vi "CONTINEOUS READ CAN.vi"(0 "interface":string(combo)="CAN0", 2 "Baudrate":u32=500000, 5 "WRITE CMD":u8[](array[numeric]) format="%.0x", 6 "Error in 2":errorcluster {"code" format="%.0x"}, 8 "Default 3":string, 9 "Default ID 1":string="20000687", 10 "CAN OPERATION":T2, 11 "WRITE AR ID":u32 format="%.0x", 13 "DataLength":u32=8, 15 "Default ID 2":string="20000688") -> (3 "ArbitrationId 2":u32 format="%.0x", 12 "Data":u8[](array[numeric]), 16 "ActualDataSize (Frames)":u32, 17 "Actual CAN Array":string[][](array[string]), 22 "CAN DATA":T1[](array[typedef]) {"Data" format="%.0x"; "ArbitrationId" format="%.0x"; "Timestamp" format="%<%I:%M:%S%3u %p\n%m/%d/%Y>T"}, 25 "can read array":u32[][](array[numeric]), 26 "Error out 2":errorcluster {"code" format="%.0x"})   [LabVIEW 2017]
uses:
  CAN_OPERATION _TYPEDEF.ctl
  <vilib>/nican/nican.llb/CanFrameTimed.ctl
  <vilib>/nican/nican.llb/xobjhandle.ctl
  <vilib>/nican/nican.llb/ncNetAttr.ctl
  d29f5f51-2dbb-4be0-bfac-dc6a67a75a0a.vi
  ef5e345f-b127-46e6-b386-8f45186839bc.vi
  bcc05463-866b-46b8-b575-a31bcf1911b9.vi
  6277f388-f3ac-4f71-9de4-5b592c734c63.vi
panel:
  out "Output Array":string[][](array[string])
  out "ActualDataSize (Frames) 2":u32
  out "ArbitrationId 3":u32 format="%.0x"
  out "initialized array":string[][](array[string])
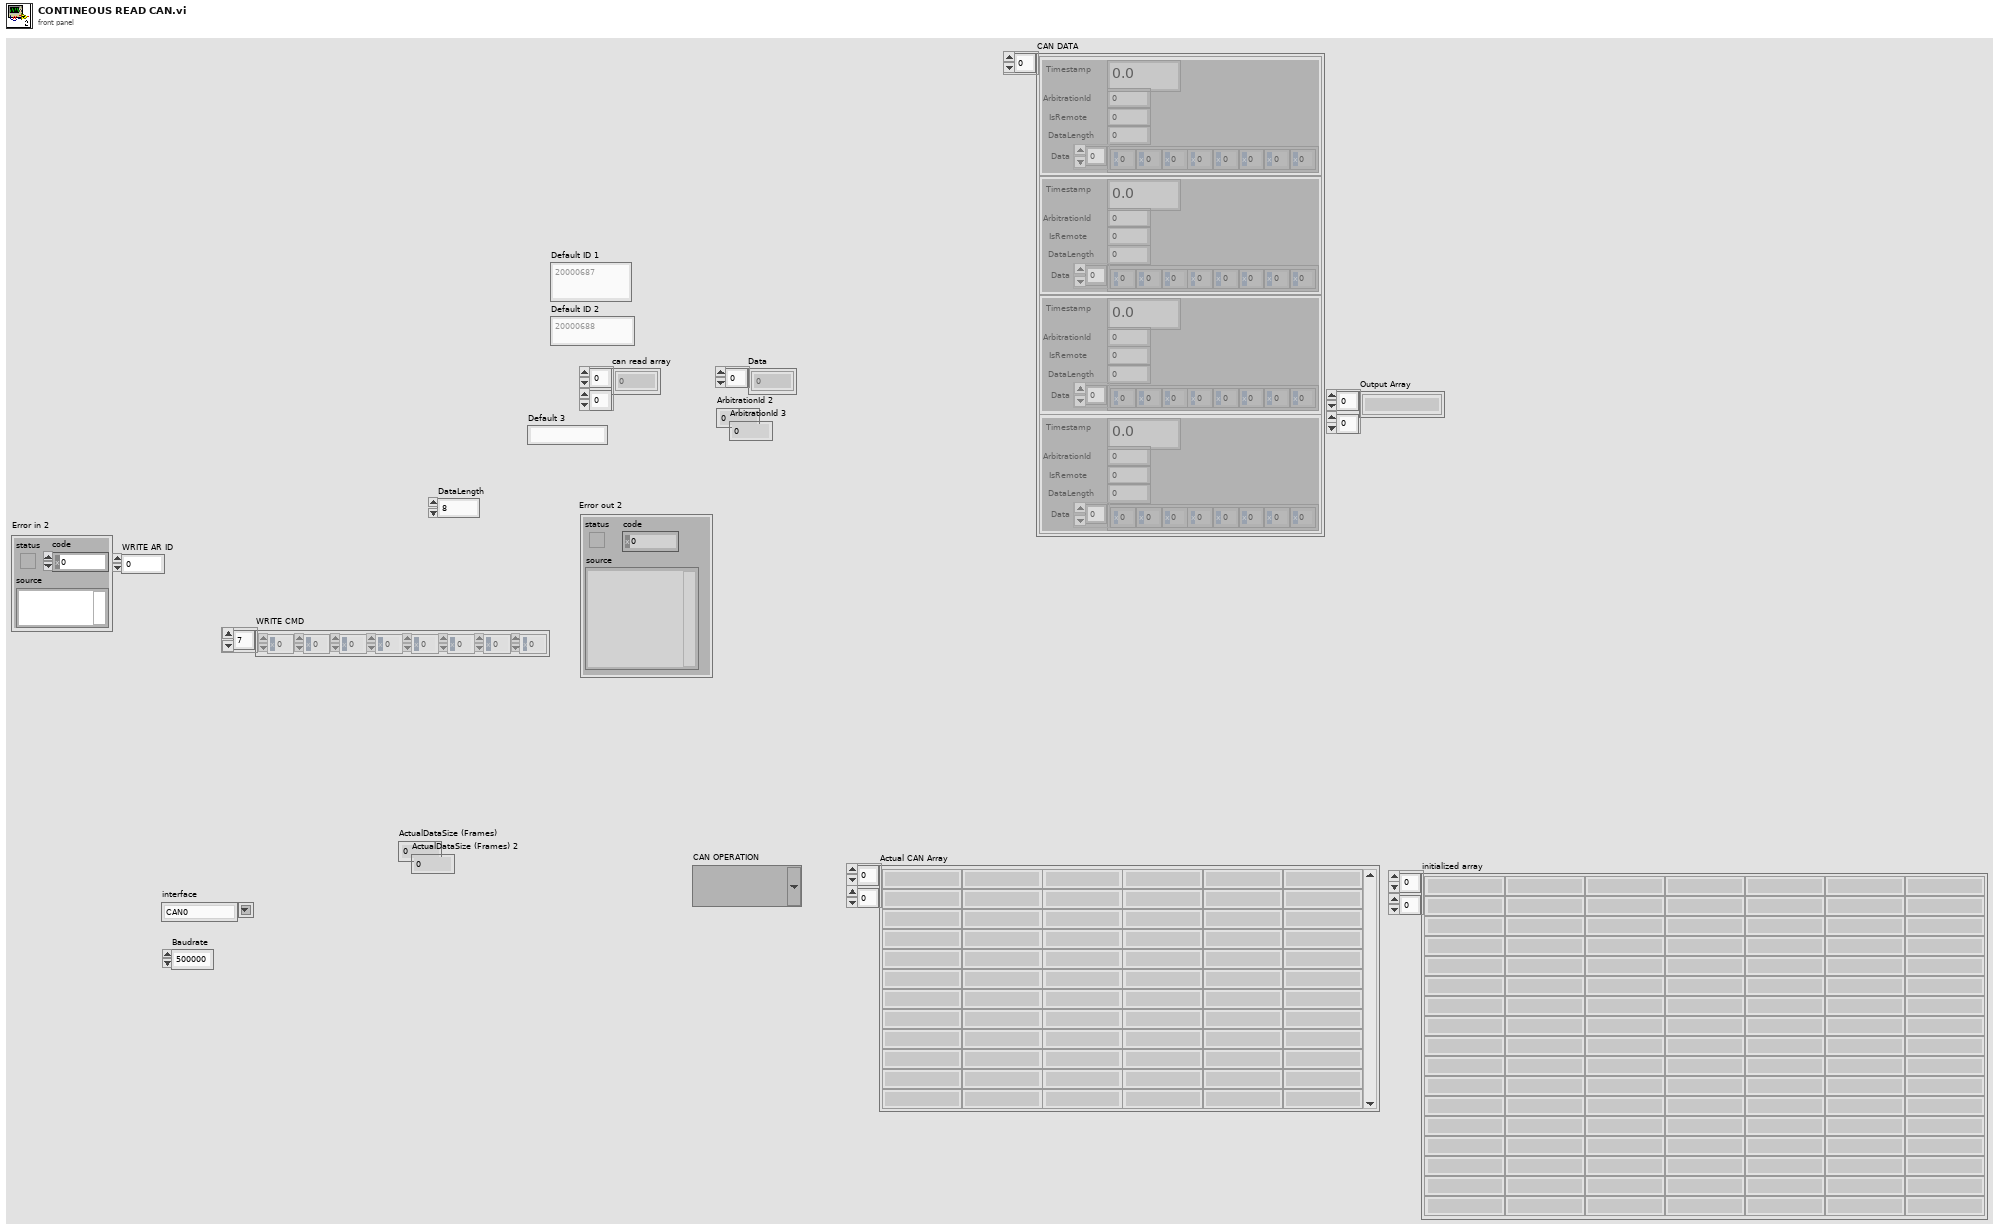
[diagram p1: front panel]
types:
  T1 = typedef "CanFrameTimed.ctl" = cluster{"Timestamp":dbl, "ArbitrationId":u32, "IsRemote":u8, "DataLength":u8, "Data":u8[]}
  T2 = typedef "CAN_OPERATION _TYPEDEF.ctl" = string
  T3 = typedef "xobjhandle.ctl" = u32
  T4 = cluster{"Baudrate":u32, "interface":string, "ObjHandle out":T3, "CAN DATA":T1[], "Data":u32[], "can read array":u32[][], "Actual CAN Array":string[][], "Default ID 1":string, "Default ID 2":string}
  T5 = typedef "ncNetAttr.ctl" = cluster{"Start On Open":enum32{"FALSE", "TRUE"}, "Baud Rate":u32, "Read Queue Length":u32, "Write Queue Length":u32, "Standard Comparator":u32, "Standard Mask":u32, "Extended Comparator":u32, "Extended Mask":u32}
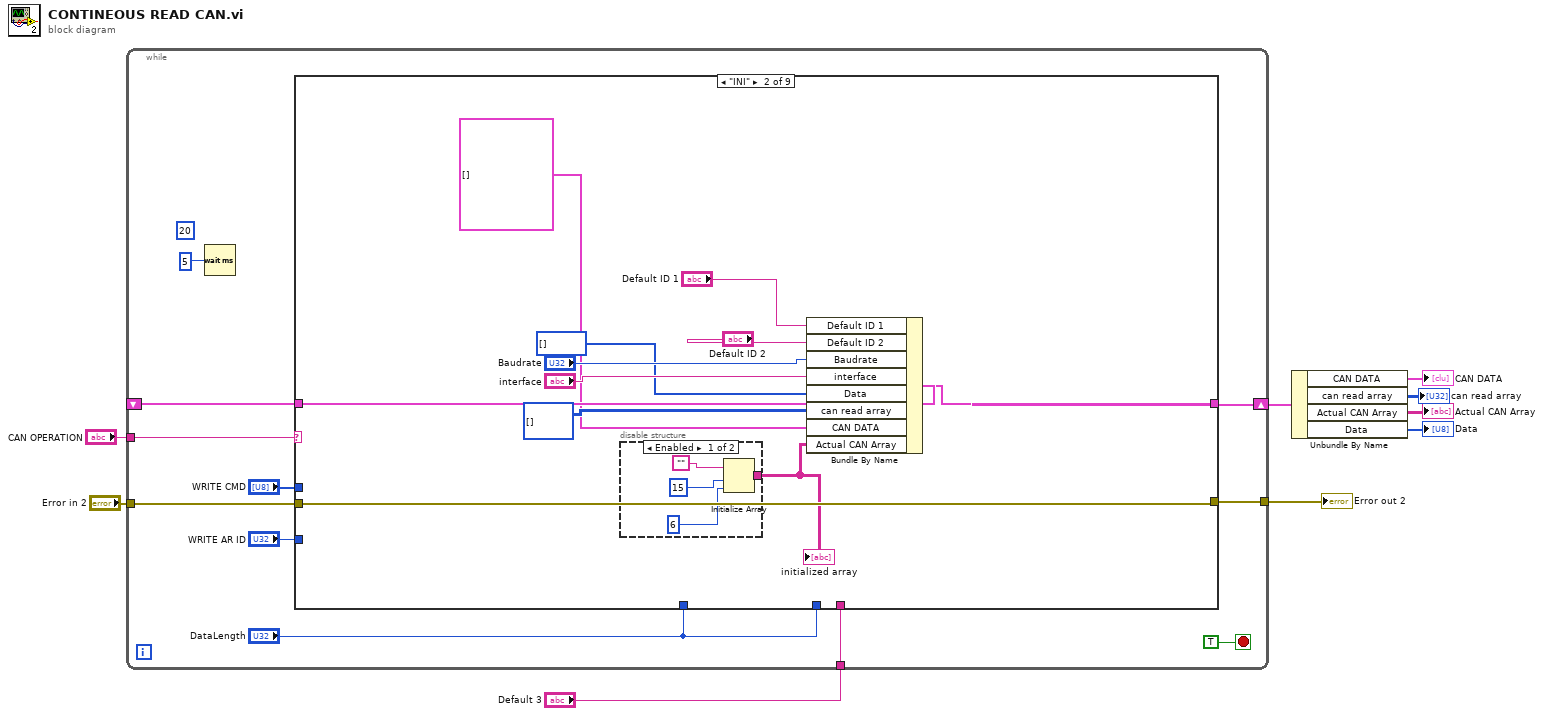
[diagram p0: block diagram]
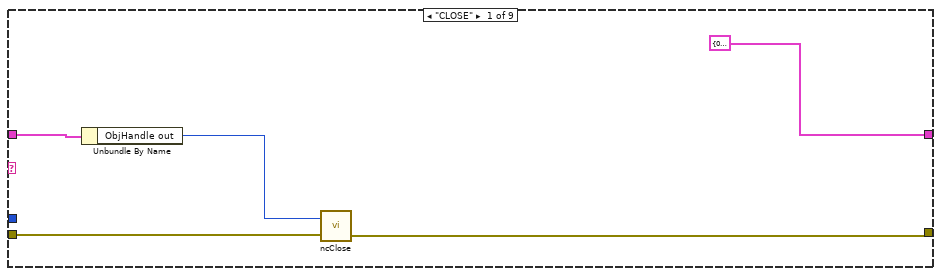
[diagram p2: hidden frame]
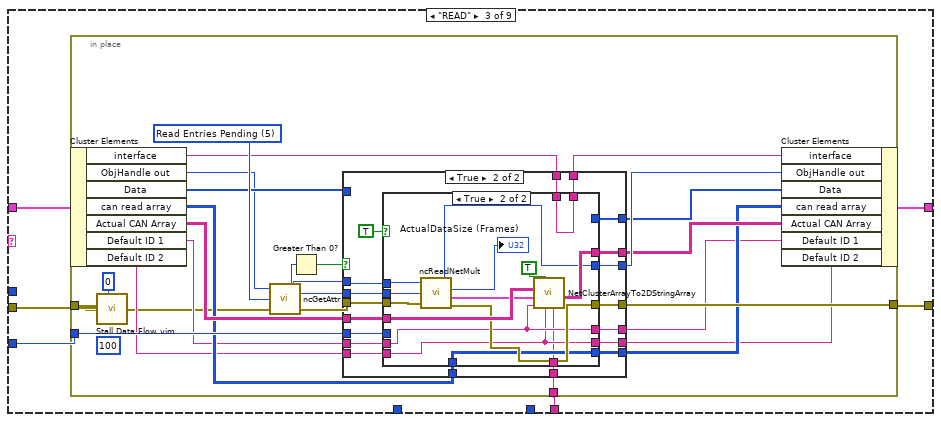
[diagram p4: hidden frame]
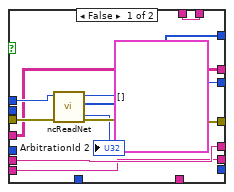
[diagram p6: hidden frame]
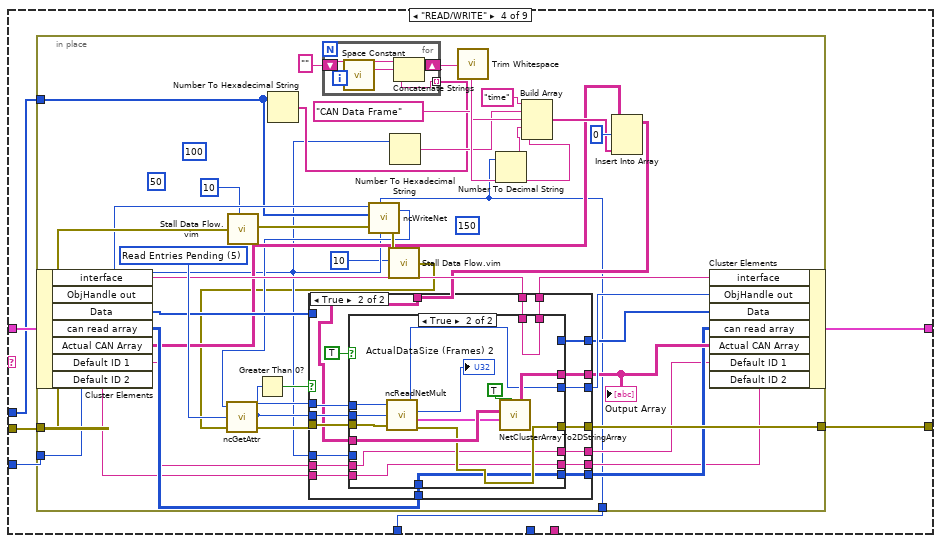
[diagram p7: hidden frame]
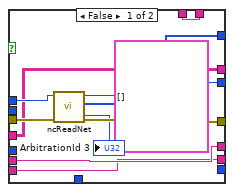
[diagram p9: hidden frame]
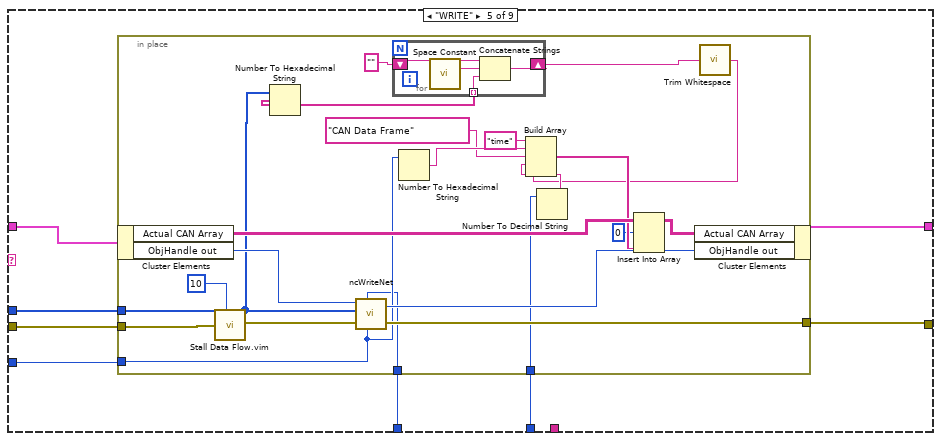
[diagram p10: hidden frame]
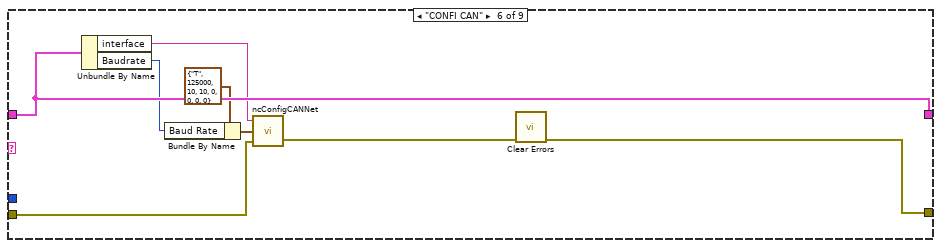
[diagram p11: hidden frame]
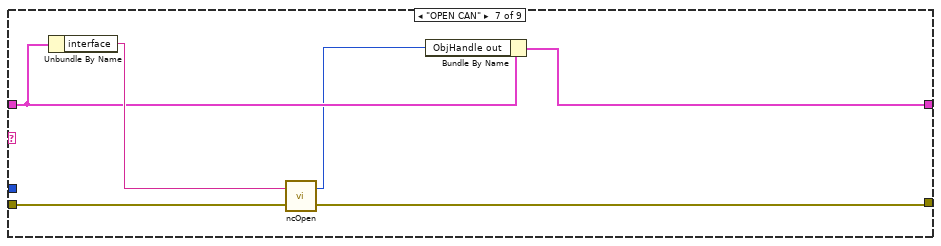
[diagram p12: hidden frame]
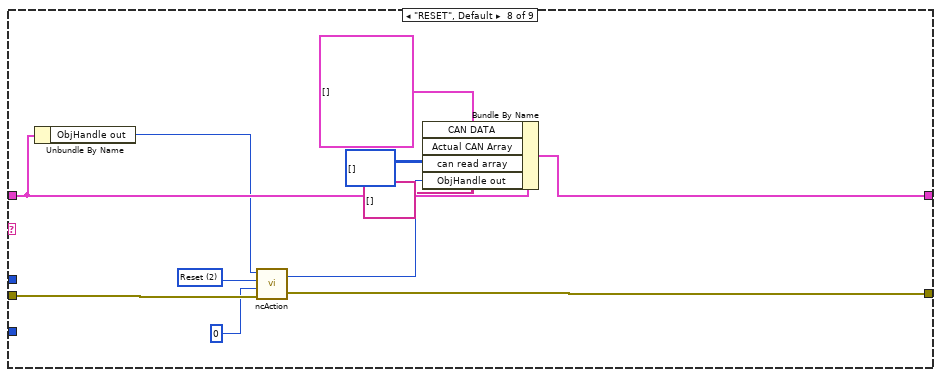
[diagram p13: hidden frame]
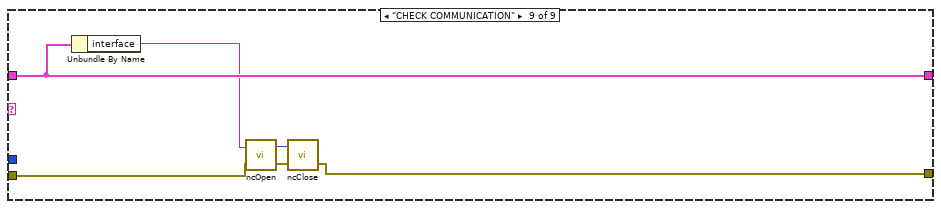
[diagram p14: hidden frame]
diagram:
  n1 = while {
    tunnel: "CAN OPERATION" -> [w20]
    tunnel: [w18] -> w2
    tunnel: "Error in 2" -> [w17]
    shift-right: [w15] -> w7
    shift-left: _ -> [w16]
    tunnel: "Default 3" -> [w10]
    stop <- TRUE stop-if-true
    (unwired) u32 20 ("millisecond multiple")
    n2 = Wait (ms)(milliseconds to wait=u32 5 ("millisecond multiple")) -> ()  [unwired: 1 out]
    n3 = case shown="\"INI\"" w20 {
      tunnel: [w24 w32 w42 w125 w229 w257 w265 w278 w285] -> w18
      tunnel: w17 -> [w25 w32 w46 w129 w230 w262 w269 w277 w282]
      tunnel: w16 -> [w23 w36 w45 w128 w225 w264 w268 w281 w284]
      tunnel: [T4 {"Baudrate"=0, "interface"="", "ObjHandle out"=0, "CAN DATA"=[], "Data"=[], "can read array"=[[710, 1, 0, 0, 0, 0, 0, 0, 0], [711, 255, 255, 255, 255, 0, 0, 0, 0], [712, 0, 0, 0, 0, 0, 0, 0, 0], [712, 0, 0, 0, 0, 0, 0, 0, 0], [720, 136, 2, 27, 96, 16, 0, 0, 0], [722, 24, 0, 0, 123, 100, 131, 12, 107], [723, 0, 0, 187, 131, 74, 4, 0, 0], [723, 0, 0, 187, 131, 74, 4, 0, 0], [725, 255, 255, 159, 111, 255, 255, 0, 0], [725, 255, 255, 159, 111, 255, 255, 0, 0], [727, 255, 255, 255, 255, 255, 29, 0, 0], [946, 144, 0, 0, 192, 192, 15, 0, 51], [1168, 197, 0, 0, 0, 0, 0, 0, 0], [1168, 197, 0, 0, 0, 0, 0, 0, 0], [1169, 0, 0, 0, 0, 0, 0, 0, 0], [1169, 0, 0, 0, 0, 0, 0, 0, 0], [1280, 0, 0, 0, 0, 0, 0, 0, 0]], "Actual CAN Array"=[["05:30:00.000", "         0", "CAN Data Frame\r\n", " 0", "No Data\r\n"], ["05:30:00.000", "         0", "CAN Data Frame\r\n", " 0", "No Data\r\n"]], "Default ID 1"="", "Default ID 2"=""} w33 w44 w127 w228 w264 w266 w280 w284] -> w15
      tunnel: "WRITE CMD" -> [_ _ _ w124 w226 _ _ _ _]
      tunnel: "WRITE AR ID" -> [_ _ w43 w126 w227 _ _ _ _]
      tunnel: "DataLength" -> [_ _ _ _ w224 _ _ _ _]
      tunnel: "DataLength" -> [_ _ _ w123 w223 _ _ _ _]
      tunnel: w10 -> [_ _ w41 _ _ _ _ _ _]
      frame "CLOSE" {
        n4 = Unbundle By Name(w23) -> ("ObjHandle out"=w22:T3)
        n5 = call <vilib>:"ncClose.vi"("Error in"=w25, "ObjHandle in"=w22) -> ("Error out"=w24:errorcluster)  [unwired: 1 in]
      }
      frame "INI" {
        n6 = disable-structure shown="Enabled" {
          disable-tunnel: [w38 _] -> w28
          frame Enabled {
            n7 = Initialize Array("", 15, 6) -> (w38:string[][])
          }
          frame Disabled {
          }
        }
        "initialized array" <- w28
        n8 = Bundle By Name(cluster=w36, "Default ID 1"="Default ID 1", "Default ID 2"="Default ID 2", "Baudrate"="Baudrate", "interface"="interface", "Data"=u8[] [], "can read array"=u32[][] [], "CAN DATA"=T1[] [], "Actual CAN Array"=w28) -> (w33:T4)
      }
      frame "READ" {
        n9 = in-place {
          in-place-border: w46 -> [w58]
          in-place-border: w43 -> [w67]
          in-place-border: [w56] -> w42
          in-place-border: w41 -> [w47]
          (unwired) u32 100 ("millisecond multiple")
          w71 = u32 5 items=["(reserved)", "Protocol Version", "Software Version", "Object State", "(reserved)", "Read Entries Pending", "Write Entries Pending", "ReadMult Size for Notification", "Listen Only?", "Self Reception?", "Transmit Error Counter", "Receive Error Counter", "Single Shot Transmit?", "Series 2 Filter Mode", "Series 2 Mask", "Series 2 Comparator", "Serial Number", "Form Factor", "Series", "Transceiver Type", "Interface Number", "Series 2 Error/Arb Capture", "Transceiver Mode", "Transceiver External Outputs", "Transceiver External Inputs", "Start Trigger Behavior", "Log Comm Warnings", "User RTSI Frame", "Transmit Mode", "Log Start Trigger?", "Timestamp Format", "Master Timebase Rate", "Virtual Bus Timing"] ("AttrId")
          n10 = in-place-cluster #1(w45) -> ("interface"=w65:string, "ObjHandle out"=w57:T3, "Data"=w61:u32[], "can read array"=w55:u32[][], "Actual CAN Array"=w62:string[][], "Default ID 1"=w53:string, "Default ID 2"=w52:string)
          n11 = call "Stall Data Flow.vim"("value in"=w58, "milliseconds to wait"=u32 0 ("millisecond multiple")) -> ("value out"=w49:errorcluster)  [unwired: 1 out]
          n12 = call <vilib>:"ncGetAttr.vi"("Error in"=w49, "AttrId"=w71, "ObjHandle in"=w57) -> ("Error out"=w59:errorcluster, "AttrValue"=w60:u32, "ObjHandle out"=w69:T3)
          n13 = Greater Than 0?(x=w60) -> (x > 0?=w70:bool)
          n14 = case shown="True" w70 {
            tunnel: w59 -> [w77 w97]
            tunnel: [w77 w86] -> w56
            tunnel: w69 -> [w78 w96]
            tunnel: [w78 w95] -> w68
            tunnel: w67 -> [_ w93]
            tunnel: [w74 w92] -> w66
            tunnel: w65 -> [w76 w91]
            tunnel: [w76 w90] -> w64
            tunnel: [w75 w89] -> w63
            tunnel: w62 -> [w75 w88]
            tunnel: w61 -> [w74 _]
            tunnel: w60 -> [_ w87]
            tunnel: w55 -> [_ w85]
            tunnel: [_ w84] -> w54
            tunnel: w53 -> [w73 w83]
            tunnel: w52 -> [w72 w82]
            tunnel: [w73 w81] -> w51
            tunnel: [w72 w80] -> w50
            tunnel: w47 -> [_ w79]
            frame False {
            }
            frame True {
              n15 = case shown="True" TRUE {
                tunnel: w97 -> [w107 w121]
                tunnel: [w106 w113] -> w86
                tunnel: w96 -> [w105 w114]
                tunnel: [w104 w117] -> w95
                tunnel: w93 -> [_ _]
                tunnel: [w102 _] -> w92
                tunnel: w91 -> [w103 w116]
                tunnel: [w103 w116] -> w90
                tunnel: [w100 w120] -> w89
                tunnel: w88 -> [w100 w119]
                tunnel: w87 -> [_ w115]
                tunnel: w85 -> [_ w111]
                tunnel: [_ w111] -> w84
                tunnel: w83 -> [w99 w110]
                tunnel: w82 -> [w98 w109]
                tunnel: [w99 w110] -> w81
                tunnel: [w98 w109] -> w80
                tunnel: w79 -> [_ w108]
                frame False {
                  (unwired) T1[] [] ("101 Array")
                  n16 = call <vilib>:"ncReadNet.vi"("ObjHandle in"=w105, "Error in"=w107) -> ("ArbitrationId"=→"ArbitrationId 2":u32, "ObjHandle out"=w104:T3, "Data"=w102:u8[], "Error out"=w106:errorcluster)  [unwired: 2 in, 3 out]
                }
                frame True {
                  n17 = call <vilib>:"ncReadNetMult.vi"("ObjHandle in"=w114, "Requested Number of Frames"=w115, "Error in"=w121) -> ("ObjHandle out"=w117:T3, "ActualDataSize (Frames)"=→"ActualDataSize (Frames)":u32, "Data"=w112:T1[], "Error out"=w113:errorcluster)
                  n18 = call <vilib>:"NetClusterArrayTo2DStringArray.vi"("Default 2"=w108, "Default 3"=w109, "Hexadecimal?"=TRUE, "Default 1"=w110, "Data from ncReadNetMult"=w112, "Input Array"=w119) -> ("Output Array"=w120:string[][])  [unwired: 5 in]
                }
              }
            }
          }
          n19 = in-place-cluster #1("interface"=w64, "ObjHandle out"=w68, "Data"=w66, "can read array"=w54, "Actual CAN Array"=w63, "Default ID 1"=w51, "Default ID 2"=w50) -> (w44:T4)
        }
      }
      frame "READ/WRITE" {
        n20 = in-place {
          in-place-border: w129 -> [w142]
          in-place-border: w126 -> [w133]
          in-place-border: [w159] -> w125
          in-place-border: w124 -> [w134]
          in-place-border: w123 -> [w132]
          (unwired) u32 150 ("milliseconds to wait")
          (unwired) u32 100 ("milliseconds to wait")
          (unwired) u32 50 ("milliseconds to wait")
          w170 = u32 5 items=["(reserved)", "Protocol Version", "Software Version", "Object State", "(reserved)", "Read Entries Pending", "Write Entries Pending", "ReadMult Size for Notification", "Listen Only?", "Self Reception?", "Transmit Error Counter", "Receive Error Counter", "Single Shot Transmit?", "Series 2 Filter Mode", "Series 2 Mask", "Series 2 Comparator", "Serial Number", "Form Factor", "Series", "Transceiver Type", "Interface Number", "Series 2 Error/Arb Capture", "Transceiver Mode", "Transceiver External Outputs", "Transceiver External Inputs", "Start Trigger Behavior", "Log Comm Warnings", "User RTSI Frame", "Transmit Mode", "Log Start Trigger?", "Timestamp Format", "Master Timebase Rate", "Virtual Bus Timing"] ("AttrId")
          n21 = in-place-cluster #2(w128) -> ("interface"=w165:string, "ObjHandle out"=w138:T3, "Data"=w162:u32[], "can read array"=w158:u32[][], "Actual CAN Array"=w139:string[][], "Default ID 1"=w156:string, "Default ID 2"=w155:string)
          n22 = call "Stall Data Flow.vim"("value in"=w142, "milliseconds to wait"=u32 10) -> ("value out"=w143:errorcluster)  [unwired: 1 out]
          n23 = Number To Hexadecimal String(2:w134) -> (0:w135:string[])  [unwired: 1 in]
          n24 = for {
            shift-right: [w173] -> w151
            shift-left: "" -> [w172]
            tunnel: w135 -> [w171] mode=indexing
            n25 = call <vilib>:"Space Constant.vi"() -> ("String"=w174:string)
            n26 = Concatenate Strings(w172, w174, w171) -> (w173:string)
          }
          n27 = call <vilib>:"ncWriteNet.vi"("ArbitrationId"=w133, "DataLength"=w132, "Error in"=w143, "Data"=w134, "ObjHandle in"=w138) -> ("Error out"=w141:errorcluster, "ObjHandle out"=w137:T3)  [unwired: 1 in]
          n28 = call "Stall Data Flow.vim"("value in"=w141, "milliseconds to wait"=u32 10) -> ("value out"=w130:errorcluster)  [unwired: 1 out]
          n29 = call <vilib>:"ncGetAttr.vi"("Error in"=w130, "AttrId"=w170, "ObjHandle in"=w137) -> ("Error out"=w160:errorcluster, "AttrValue"=w161:u32, "ObjHandle out"=w168:T3)
          n30 = Greater Than 0?(x=w161) -> (x > 0?=w169:bool)
          n31 = Number To Hexadecimal String(2:w133) -> (0:w144:string)  [unwired: 1 in]
          n32 = call <vilib>:"Trim Whitespace.vi"("string"=w151) -> ("trimmed string"=w152:string)  [unwired: 1 in]
          n33 = Number To Decimal String(number=w132) -> (decimal integer string=w145:string)  [unwired: 1 in]
          n34 = Build Array("time" ("element"), w144, "CAN Data Frame", w145, w152) -> (w148:string[])
          n35 = Insert Into Array(array=w139, index (row)=0, new element=w148) -> (w140:string[][])  [unwired: 1 in]
          n36 = case shown="True" w169 {
            tunnel: w160 -> [w179 w198]
            tunnel: [w179 w188] -> w159
            tunnel: w168 -> [w180 w197]
            tunnel: [w180 w196] -> w167
            tunnel: w133 -> [_ w194]
            tunnel: [w177 w193] -> w166
            tunnel: w165 -> [w178 w192]
            tunnel: [w178 w191] -> w164
            tunnel: [_ w190] -> w163
            tunnel: w162 -> [w177 _]
            tunnel: w161 -> [_ w189]
            tunnel: w158 -> [_ w187]
            tunnel: [_ w186] -> w157
            tunnel: w156 -> [w176 w185]
            tunnel: w155 -> [w175 w184]
            tunnel: [w176 w183] -> w154
            tunnel: [w175 w182] -> w153
            tunnel: w140 -> [_ w181]
            frame False {
            }
            frame True {
              n37 = case shown="True" TRUE {
                tunnel: w198 -> [w208 w221]
                tunnel: [w207 w213] -> w188
                tunnel: w197 -> [w206 w214]
                tunnel: [w205 w217] -> w196
                tunnel: w194 -> [_ _]
                tunnel: [w203 _] -> w193
                tunnel: w192 -> [w204 w216]
                tunnel: [w204 w216] -> w191
                tunnel: [w201 w220] -> w190
                tunnel: w181 -> [w201 w219]
                tunnel: w189 -> [_ w215]
                tunnel: w187 -> [_ w211]
                tunnel: [_ w211] -> w186
                tunnel: w185 -> [w200 w210]
                tunnel: w184 -> [w199 w209]
                tunnel: [w200 w210] -> w183
                tunnel: [w199 w209] -> w182
                frame False {
                  (unwired) T1[] [] ("101 Array")
                  n38 = call <vilib>:"ncReadNet.vi"("ObjHandle in"=w206, "Error in"=w208) -> ("ArbitrationId"=→"ArbitrationId 3":u32, "ObjHandle out"=w205:T3, "Data"=w203:u8[], "Error out"=w207:errorcluster)  [unwired: 2 in, 3 out]
                }
                frame True {
                  n39 = call <vilib>:"ncReadNetMult.vi"("ObjHandle in"=w214, "Requested Number of Frames"=w215, "Error in"=w221) -> ("ObjHandle out"=w217:T3, "ActualDataSize (Frames)"=→"ActualDataSize (Frames) 2":u32, "Data"=w212:T1[], "Error out"=w213:errorcluster)
                  n40 = call <vilib>:"NetClusterArrayTo2DStringArray.vi"("Hexadecimal?"=TRUE, "Data from ncReadNetMult"=w212, "Input Array"=w219) -> ("Output Array"=w220:string[][])  [unwired: 8 in]
                }
              }
            }
          }
          "Output Array" <- w163
          n41 = in-place-cluster #2("interface"=w164, "ObjHandle out"=w167, "Data"=w166, "can read array"=w157, "Actual CAN Array"=w163, "Default ID 1"=w154, "Default ID 2"=w153) -> (w127:T4)
        }
      }
      frame "WRITE" {
        n42 = in-place {
          in-place-border: w230 -> [w252]
          in-place-border: [w251] -> w229
          in-place-border: w226 -> [w240]
          in-place-border: w227 -> [w241]
          in-place-border: w224 -> [w232]
          in-place-border: w223 -> [w231]
          n43 = in-place-cluster #3(w225) -> ("Actual CAN Array"=w242:string[][], "ObjHandle out"=w250:T3)
          n44 = call "Stall Data Flow.vim"("value in"=w252, "milliseconds to wait"=u32 10) -> ("value out"=w248:errorcluster)  [unwired: 1 out]
          n45 = Number To Hexadecimal String(2:w240) -> (0:w239:string[])  [unwired: 1 in]
          n46 = call <vilib>:"ncWriteNet.vi"("ArbitrationId"=w241, "DataLength"=w231, "Error in"=w248, "Data"=w240, "ObjHandle in"=w250) -> ("Error out"=w251:errorcluster, "ObjHandle out"=w249:T3)  [unwired: 1 in]
          n47 = for {
            shift-right: [w255] -> w234
            shift-left: "" -> [w254]
            tunnel: w239 -> [w253] mode=indexing
            n48 = call <vilib>:"Space Constant.vi"() -> ("String"=w256:string)
            n49 = Concatenate Strings(w254, w256, w253) -> (w255:string)
          }
          n50 = Number To Hexadecimal String(2:w241) -> (0:w246:string)  [unwired: 1 in]
          n51 = Number To Decimal String(number=w232) -> (decimal integer string=w245:string)  [unwired: 1 in]
          n52 = call <vilib>:"Trim Whitespace.vi"("string"=w234) -> ("trimmed string"=w233:string)  [unwired: 1 in]
          n53 = Build Array("time" ("element"), w246, "CAN Data Frame", w245, w233) -> (w238:string[])
          n54 = Insert Into Array(array=w242, index (row)=0, new element=w238) -> (w237:string[][])  [unwired: 1 in]
          n55 = in-place-cluster #3("Actual CAN Array"=w237, "ObjHandle out"=w249) -> (w228:T4)
        }
      }
      frame "CONFI CAN" {
        n56 = Unbundle By Name(w264) -> ("interface"=w263:string, "Baudrate"=w258:u32)
        n57 = Bundle By Name(cluster=T5 {"Start On Open"=enum."TRUE", "Baud Rate"=125000, "Read Queue Length"=10, "Write Queue Length"=10, "Standard Comparator"=0, "Standard Mask"=0, "Extended Comparator"=0, "Extended Mask"=0} ("CAN Network Interface Config"), "Baud Rate"=w258) -> (w259:T5)
        n58 = call <vilib>:"ncConfigCANNet.vi"("Error in"=w262, "CAN Network Interface Config"=w259, "ObjName"=w263) -> ("Error out"=w261:errorcluster)  [unwired: 2 in]
        n59 = call <vilib>:"Clear Errors.vi"("error in (no error)"=w261) -> ("error out"=w257:errorcluster)  [unwired: 5 in, 1 out]
      }
      frame "OPEN CAN" {
        n60 = Unbundle By Name(w268) -> ("interface"=w270:string)
        n61 = call <vilib>:"ncOpen.vi"("Error in"=w269, "ObjName"=w270) -> ("Error out"=w265:errorcluster, "ObjHandle out"=w267:T3)
        n62 = Bundle By Name(cluster=w268, "ObjHandle out"=w267) -> (w266:T4)
      }
      frame "RESET", Default {
        w279 = u32 2 items=["Start", "Stop", "Reset", "Output on RTSI line"] ("Opcode")
        n63 = Unbundle By Name(w281) -> ("ObjHandle out"=w276:T3)
        n64 = call <vilib>:"ncAction.vi"("Error in"=w277, "Param"=u32 0, "Opcode"=w279, "ObjHandle in"=w276) -> ("Error out"=w278:errorcluster, "ObjHandle out"=w275:T3)
        n65 = Bundle By Name(cluster=w281, "CAN DATA"=T1[] [], "Actual CAN Array"=string[][] [], "can read array"=u32[][] [], "ObjHandle out"=w275) -> (w280:T4)
      }
      frame "CHECK COMMUNICATION" {
        n66 = Unbundle By Name(w284) -> ("interface"=w283:string)
        n67 = call <vilib>:"ncOpen.vi"("Error in"=w282, "ObjName"=w283) -> ("Error out"=w287:errorcluster, "ObjHandle out"=w286:T3)
        n68 = call <vilib>:"ncClose.vi"("Error in"=w287, "ObjHandle in"=w286) -> ("Error out"=w285:errorcluster)  [unwired: 1 in]
      }
    }
  }
  "Error out 2" <- w2
  n69 = Unbundle By Name(w7) -> ("CAN DATA"=→"CAN DATA":T1[], "can read array"=→"can read array":u32[][], "Actual CAN Array"=→"Actual CAN Array":string[][], "Data"=→"Data":u32[])
